vi "ex_needTimeChannelNow.vi"(1 "index":i32, 2 "x_columns":u16) -> (0 "need time channel NOW !!!!":bool)   [LabVIEW 2017]
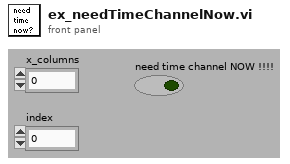
[diagram p1: front panel]
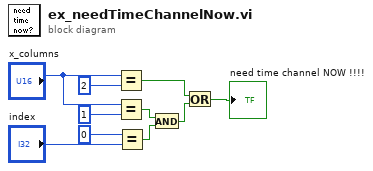
[diagram p0: block diagram]
diagram:
  n1 = Equal?(x="x_columns", y=u16 2) -> (x = y?=w9:bool)
  n2 = Equal?(x="x_columns", y=u16 1) -> (x = y?=w6:bool)
  n3 = Equal?(x=0, y="index") -> (x = y?=w7:bool)
  n4 = And(x=w6, y=w7) -> (x .and. y?=w8:bool)
  n5 = Or(x=w9, y=w8) -> (x .or. y?=→"need time channel NOW !!!!":bool)
